vi "Program Control.vi"(0 "Display State In":T1={"Measure ?"=[], "Direction"=[], "Loop ?"={"Start"=0, "Finish"=2}, "Storage Location"=[], "Show Current Location"=FALSE, "Current Location"=0, "Show y=0"=FALSE, "Program"=[], "Index"=0, "Average During Loop ?"=FALSE, "# of Loops"=1, "Loop Control"={0, 2}, "Units"="", "Digits"=0, "Significant Figures (F) or DP (T)"=FALSE, "Rate Mode"=FALSE, "Current Y value"=0.0, "Initial Value"=0.0} {"# of Loops" min=1 step=1; "Index" min=0 step=1; "Program"."Step" min=0.001 max=80.0 step=0.001 format="%.2f"; "Program"."Target" format="%.2f"}, 1 "Steps":dbl[](array[numeric]), 5 "Start":dbl, 7 "Targets":dbl[](array[numeric]), 9 "Container State":T2, 11 "error in (no error)":errorcluster, 12 "Measure?":bool[](array[boolean])) -> (4 "Display State Out":T1={"Measure ?"=[], "Direction"=[], "Loop ?"={"Start"=0, "Finish"=2}, "Storage Location"=[], "Show Current Location"=FALSE, "Current Location"=0, "Show y=0"=FALSE, "Program"=[], "Index"=0, "Average During Loop ?"=FALSE, "# of Loops"=1, "Loop Control"={0, 2}, "Units"="", "Digits"=0, "Significant Figures (F) or DP (T)"=FALSE, "Rate Mode"=FALSE, "Current Y value"=0.0, "Initial Value"=0.0} {"# of Loops" min=1 step=1; "Index" min=0 step=1; "Program"."Step" min=0.001 max=80.0 step=0.001 format="%.2f"; "Program"."Target" format="%.2f"}, 15 "error out":errorcluster)   [LabVIEW 2018, in "Multi Segment Waveform.xctl"]
uses:
  Multi Segment Waveform.xctl
  <vilib>/_xctls/Container State.ctl
  State.ctl
  <vilib>/_xctls/XControlSupport.lvlib
panel:
  # "Add Controls & Indicators that form the parameters of the method here. Hook them to the connector pane. Do not delete the controls & indicators that are already hooked to the connector pane.\n \nTo setup the parameters  for this method, right click on this item in the Project Tree & select \"Configure Method...\"."
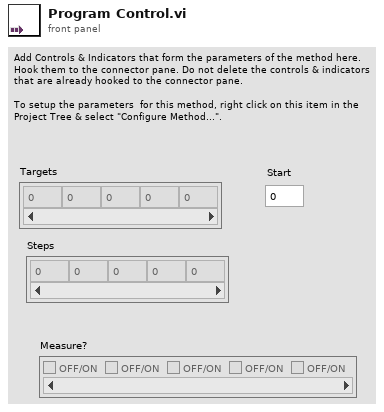
[diagram p1: front panel]
types:
  T1 = typedef "Multi Segment Waveform.xctl/State.ctl" = cluster{"Measure ?":bool[], "Direction":bool[], "Loop ?":cluster{"Start":i32, "Finish":i32}, "Storage Location":i32[], "Show Current Location":bool, "Current Location":i32, "Show y=0":bool, "Program":cluster{"Target":dbl, "Step":dbl, "Measure ?":bool}[], "Index":i32, "Average During Loop ?":bool, "# of Loops":u32, "Loop Control":cluster{i32, i32}, "Units":string, "Digits":i32, "Significant Figures (F) or DP (T)":bool, "Rate Mode":bool, "Current Y value":dbl, "Initial Value":dbl}
  T2 = typedef "XControlSupport.lvlib/Container State.ctl" = cluster{"Indicator?":bool, "Run Mode?":bool, " Refnum":refnum<vi>}
  T3 = cluster{"Numeric":dbl, "Numeric":dbl, "Boolean":bool}[]
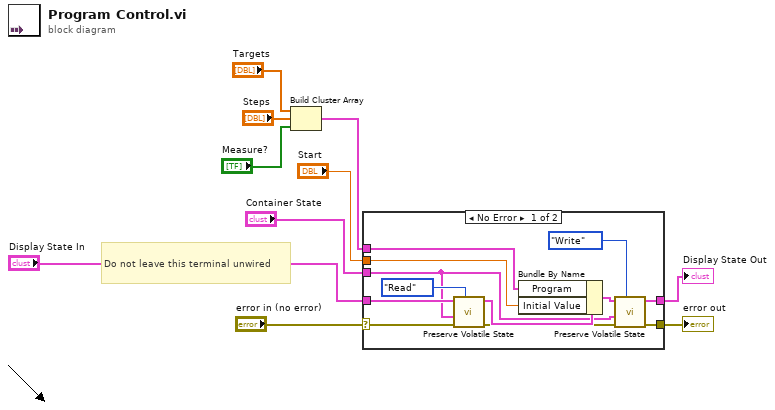
[diagram p0: block diagram]
diagram:
  # "Do not leave this terminal unwired"
  n1 = Build Cluster Array("Targets", "Steps", "Measure?") -> (w2:T3)
  n2 = case shown="No Error" "error in (no error)" {
    selector: "error in (no error)" -> [w20 w24]
    tunnel: "Display State In" -> [w22 w23]
    tunnel: "Container State" -> [w17 _]
    tunnel: [w14 w24] -> w3
    tunnel: [w13 w23] -> w5
    tunnel: w2 -> [w12 _]
    tunnel: "Start" -> [w11 _]
    frame No Error {
      n3 = call "Preserve Volatile State.vi"("Operation"=enum16{"Read", "Write", "Update From Data"}."Read", "error in (no error)"=w20, "Container State"=w17, "Waveform State In"=w22) -> ("error out"=w16:errorcluster, "Waveform State Out"=w19:T1)  [unwired: 1 in, 5 out]
      n4 = Bundle By Name(cluster=w19, "Program"=w12, "Initial Value"=w11) -> (w18:T1)
      n5 = call "Preserve Volatile State.vi"("Operation"=enum16{"Read", "Write", "Update From Data"}."Write", "error in (no error)"=w16, "Container State"=w17, "Waveform State In"=w18) -> ("error out"=w14:errorcluster, "Waveform State Out"=w13:T1)  [unwired: 1 in, 5 out]
    }
    frame Error {
    }
  }
  "Display State Out" <- w5
  "error out" <- w3
